vi "setTemperature.vi"(6 "Channel":i32, 8 "error in (no error)":errorcluster, 9 "Rate (K/min)":dbl, 10 "Temperature (K)":dbl, 11 "Instrument.Cryostat in":refnum<class "Instrument.Cryostat.lvclass">) -> (0 "error out":errorcluster, 3 "Instrument.Cryostat out":refnum<class "Instrument.Cryostat.lvclass">)   [LabVIEW 2019, in "Instrument.Cryostat.lvclass"]
uses:
  Instrument.Cryostat.lvclass
  C:/Users/patrick/Documents/GitHub/Instrument-Framework/lvsrc/Instrument/Instrument.lvclass
  Typedefs/setTemperature--cluster.ctl
  Instrument/Instrument.lvclass/Instrument.ctl
  842ad4d8-f68b-4c23-9e9f-32f793385417.vi
  842ad4d8-f68b-4c23-9e9f-32f793385417.vi/edf7c4b0-a978-4818-a2ab-74c5d28f1262.vi
  842ad4d8-f68b-4c23-9e9f-32f793385417.vi/8d680e1c-5661-4cd1-8d70-5899a69fc731.vi
  Instrument/Private/Get Client Type.vi
  842ad4d8-f68b-4c23-9e9f-32f793385417.vi/edf7c4b0-a978-4818-a2ab-74c5d28f1262.vi/4576bc7c-8f69-48b8-b0d8-7ab47e2b6100.vi
  842ad4d8-f68b-4c23-9e9f-32f793385417.vi/edf7c4b0-a978-4818-a2ab-74c5d28f1262.vi/d509161e-6b2e-4507-8b95-380cbea5b3b8.vi
  Instrument/Private/Set Dependencies.vi
  842ad4d8-f68b-4c23-9e9f-32f793385417.vi/8d680e1c-5661-4cd1-8d70-5899a69fc731.vi/267c46a6-5146-4dba-8066-e2aed85009e6.vi
  842ad4d8-f68b-4c23-9e9f-32f793385417.vi/8d680e1c-5661-4cd1-8d70-5899a69fc731.vi/3d23412b-6c21-499e-8eac-e96b59108135.vi
  842ad4d8-f68b-4c23-9e9f-32f793385417.vi/8d680e1c-5661-4cd1-8d70-5899a69fc731.vi/508fc9dc-f157-44b8-8779-4da7f6c28100.vi
  842ad4d8-f68b-4c23-9e9f-32f793385417.vi/edf7c4b0-a978-4818-a2ab-74c5d28f1262.vi/d509161e-6b2e-4507-8b95-380cbea5b3b8.vi/7654db8a-0638-4ea4-a87a-3933e57c9943.vi
  842ad4d8-f68b-4c23-9e9f-32f793385417.vi/edf7c4b0-a978-4818-a2ab-74c5d28f1262.vi/d509161e-6b2e-4507-8b95-380cbea5b3b8.vi/2cfa170f-6c3d-4e10-b8d0-4a1db59c58c2.vi
  842ad4d8-f68b-4c23-9e9f-32f793385417.vi/8d680e1c-5661-4cd1-8d70-5899a69fc731.vi/3d23412b-6c21-499e-8eac-e96b59108135.vi/bf3d8fb9-81db-4e71-8b15-51eebc0546e2.vi
  842ad4d8-f68b-4c23-9e9f-32f793385417.vi/8d680e1c-5661-4cd1-8d70-5899a69fc731.vi/3d23412b-6c21-499e-8eac-e96b59108135.vi/000b6ca1-1b96-4bf5-b82c-e0fd6fc4fe97.vi
  842ad4d8-f68b-4c23-9e9f-32f793385417.vi/8d680e1c-5661-4cd1-8d70-5899a69fc731.vi/508fc9dc-f157-44b8-8779-4da7f6c28100.vi/c64594e2-7ff0-4a20-b4d9-1d3fee304614.vi
  842ad4d8-f68b-4c23-9e9f-32f793385417.vi/8d680e1c-5661-4cd1-8d70-5899a69fc731.vi/508fc9dc-f157-44b8-8779-4da7f6c28100.vi/c3cf7e84-3709-4801-96af-ff444011670f.vi
  Instrument/Private/Get RC Connection Status.vi
  Instrument/Private/Get Dependencies.vi
  <userlib>/LevyLab/RemoteControl/API/Send and Receive.vi
  <vilib>/Utility/Data Type/Get Type Information.vi
  <vilib>/JDP Science/JSONtext/JSON text to Variant.vi
  Instrument/API/Instrument.GetPublicEvents.vi
  <vilib>/JDP Science/JSONtext/Variant to JSON Text.vi
  <vilib>/National Instruments/GUID Generator/Guid Generator.vi
  Instrument/API/Instrument.sendMessageToProcess.vi
  Instrument/Private/Instrument.MessageFromProcess.EventStructure.vi
  <vilib>/JDP Science/JSONtext/LVClass Serializer/JSONtext LVClass Serializer.lvclass
  Instrument/Instrument.lvclass
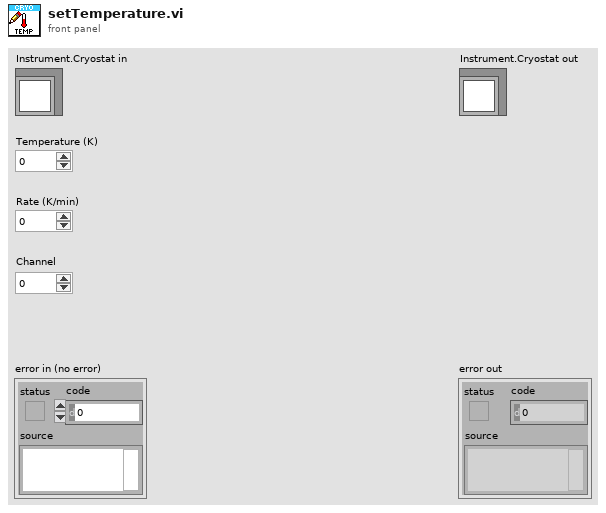
[diagram p1: front panel]
types:
  T1 = typedef "Instrument.Cryostat.lvclass/setTemperature--cluster.ctl" = cluster{"Temperature (K)":dbl, "Rate (K/min)":dbl, "Channel":i32}
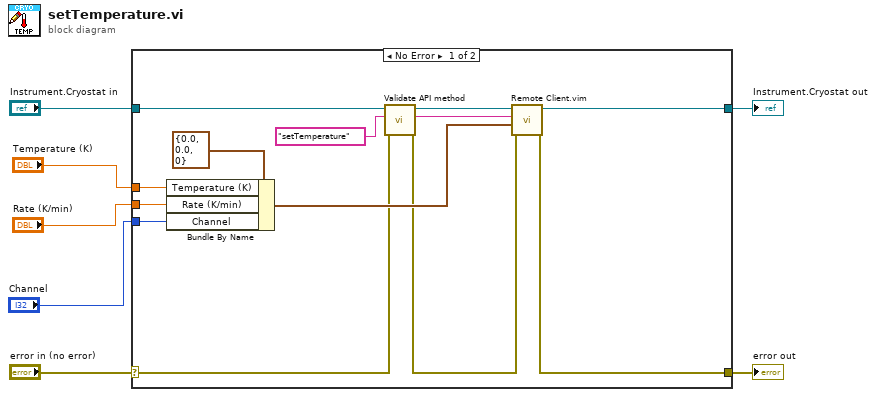
[diagram p0: block diagram]
diagram:
  n1 = case shown="No Error" "error in (no error)" {
    selector: "error in (no error)" -> [w10 w22]
    tunnel: [w9 w22] -> w6
    tunnel: [w12 w21] -> w4
    tunnel: "Instrument.Cryostat in" -> [w11 w21]
    tunnel: "Temperature (K)" -> [w19 _]
    tunnel: "Rate (K/min)" -> [w18 _]
    tunnel: "Channel" -> [w17 _]
    frame No Error {
      n2 = Bundle By Name(cluster=T1 {"Temperature (K)"=0.0, "Rate (K/min)"=0.0, "Channel"=0} ("Set Temperature"), "Temperature (K)"=w19, "Rate (K/min)"=w18, "Channel"=w17) -> (w14:T1)
      n3 = call "Validate API method.vi"("error in (no error)"=w10, "command in"="setTemperature" ("error message (\"\")"), "Instrument in"=w11) -> ("error out"=w8:errorcluster, "command out"=w15:string, "Instrument out"=w13:refnum<class "Instrument.Cryostat.lvclass">)  [unwired: 6 in]
      n4 = call "Remote Client.vim"("error in (no error)"=w8, "params"=w14, "method"=w15, "Instrument in"=w13) -> ("error out"=w9:errorcluster, "Instrument out"=w12:refnum<class "Instrument.Cryostat.lvclass">)  [unwired: 4 in, 2 out]
    }
    frame Error {
    }
  }
  "error out" <- w6
  "Instrument.Cryostat out" <- w4
